vi "cw_1.vi"() -> ()   [LabVIEW 2022 SP3]
panel:
  out "x-y*floor(x/y) 2":dbl
  out "x-y*floor(x/y)":dbl
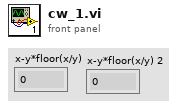
[diagram p1: front panel]
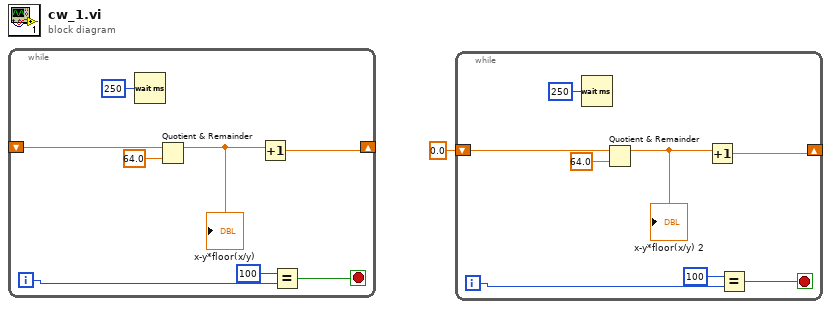
[diagram p0: block diagram]
diagram:
  n1 = while {
    shift-right: [w5] -> _
    shift-left: _ -> [w4]
    i -> [w8]
    stop <- w7 stop-if-true
    n2 = Wait (ms)(milliseconds to wait=u32 250) -> ()  [unwired: 1 out]
    n3 = Quotient & Remainder(x=w4, y=64.0) -> (x-y*floor(x/y)=w6:dbl)  [unwired: 1 out]
    "x-y*floor(x/y)" <- w6
    n4 = Increment(x=w6) -> (x+1=w5:dbl)
    n5 = Equal?(x=100, y=w8) -> (x = y?=w7:bool)
  }
  n6 = while {
    shift-right: [w13] -> _
    shift-left: 0.0 -> [w12]
    i -> [w16]
    stop <- w15 stop-if-true
    n7 = Wait (ms)(milliseconds to wait=u32 250) -> ()  [unwired: 1 out]
    n8 = Quotient & Remainder(x=w12, y=64.0) -> (x-y*floor(x/y)=w14:dbl)  [unwired: 1 out]
    "x-y*floor(x/y) 2" <- w14
    n9 = Increment(x=w14) -> (x+1=w13:dbl)
    n10 = Equal?(x=100, y=w16) -> (x = y?=w15:bool)
  }
